vi "Execute.UI.Running.vi"(8 "error in (no error)":errorcluster, 11 "Cluster":T1={"NIVS.BaseLogPath"=path "", "NIVS.SystemDefinitionFile"=path "", "NIVS.Events"={"SequenceEvent"=refnum, "SystemChangeEvent"=refnum, "WorkspaceEvent"=refnum}, "NIVS.SequenceState"=enum."Idle", "NIVS.GatewayIPAddress"="", "NIVS.DataLogSpecRef"=refnum, "NIVS.DataLogManagerRef"=refnum, "NIVS.LogSessionGUID"="", "NIVS.WorkspaceManager"=refnum, "NIVS.Deployed"=FALSE, "NIVS.ProfileRef"=refnum, "NIVS.ProfileCallback"=refnum, "NIVS.SystemStateRefs"={"CustDatRef"=refnum, "EvtRef"=refnum}, "UI.Abort"=refnum, "UI.Pause"=refnum, "UI.EnableLogging"=refnum, "UI.Start"=refnum, "UI.LogChannels"=refnum, "UI.StartIteration"=refnum, "UI.StartStep"=refnum, "UI.Sequence"=refnum, "UI.PreviewMode"=refnum, "UI.Graph"=refnum, "UI.BaseFileName"=refnum, "UI.Profiles"=refnum, "UI.CurrentStep"=refnum, "UI.CurrentIteration"=refnum, "UI.TotalIterations"=refnum, "Sequence.AbortChannel"="", "Sequence.StepInfoChannel"="", "Sequence.Iterations"=0, "Sequence.IterationInfoChannel"="", "Sequence.#ofColumns"=0, "Events.State"=refnum, "Events.Test Result"=refnum, "Events.Progress"=refnum, "INI.Settings"={"Build Location"=path "C:/Simple Sequence Editor/SequenceRepo", "LoggingLocation"=path ""}, "UI.Skip"=refnum, "Sequence.SkipChannel"="", "Restart.Path"=path "", "UI.Duration"=refnum, "Sequence.DurationChannel"=""}) -> (0 "error out":errorcluster)   [LabVIEW 2013, in "Simple Sequence Tools - Execution.lvlib"]
uses:
  Simple Sequence Tools - Execution.lvlib
  Types/Main.StateVariables.ctl
  Types/Execute.UserEventRefs.ctl
  <vilib>/NI Veristand/Execution/Workspace/SystemStateRegEventRef.ctl
  Types/Execution.SequenceState.ctl
  <vilib>/NI Veristand/Execution/DataLogging/DataLoggingSpecification Ref.ctl
  NationalInstruments.VeriStand.ClientAPI
  <vilib>/NI Veristand/Execution/DataLogging/IDataLogging Ref.ctl
  <vilib>/NI Veristand/Execution/Workspace/WorkspaceAPI.ctl
  NationalInstruments.VeriStand.RealTimeSequenceDefinitionApi
  <vilib>/NI Veristand/Execution/Workspace/SystemStateEventRef.ctl
  Shared/Types/INI.Settings
  <vilib>/NI Veristand/Execution/Workspace/NI_VS Workspace ExecutionAPI.lvlib
  <vilib>/NI Veristand/Execution/DataLogging/NI_VS Data Logging API.lvlib
  Shared/Simple Sequence Tools - Shared.lvlib
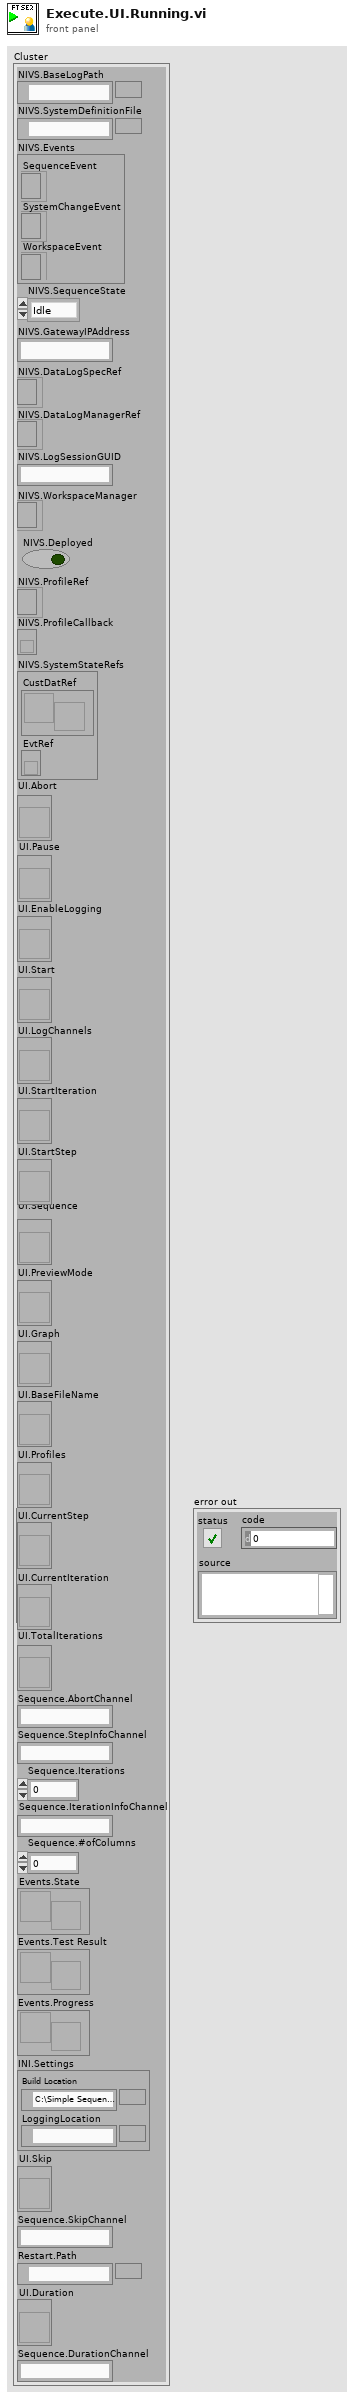
[diagram p1: front panel]
types:
  T1 = typedef "Simple Sequence Tools - Execution.lvlib/Main.StateVariables.ctl" = cluster{"NIVS.BaseLogPath":path, "NIVS.SystemDefinitionFile":path, "NIVS.Events":T2, "NIVS.SequenceState":T4, "NIVS.GatewayIPAddress":string, "NIVS.DataLogSpecRef":T5, "NIVS.DataLogManagerRef":T6, "NIVS.LogSessionGUID":string, "NIVS.WorkspaceManager":T7, "NIVS.Deployed":bool, "NIVS.ProfileRef":refnum<k24>, "NIVS.ProfileCallback":refnum<k27>, "NIVS.SystemStateRefs":T8, "UI.Abort":refnum<vi>, "UI.Pause":refnum<vi>, "UI.EnableLogging":refnum<vi>, "UI.Start":refnum<vi>, "UI.LogChannels":refnum<vi>, "UI.StartIteration":refnum<vi>, "UI.StartStep":refnum<vi>, "UI.Sequence":refnum<vi>, "UI.PreviewMode":refnum<vi>, "UI.Graph":refnum<vi>, "UI.BaseFileName":refnum<vi>, "UI.Profiles":refnum<vi>, "UI.CurrentStep":refnum<vi>, "UI.CurrentIteration":refnum<vi>, "UI.TotalIterations":refnum<vi>, "Sequence.AbortChannel":string, "Sequence.StepInfoChannel":string, "Sequence.Iterations":u32, "Sequence.IterationInfoChannel":string, "Sequence.#ofColumns":i32, "Events.State":refnum<user-event>, "Events.Test Result":refnum<user-event>, "Events.Progress":refnum<user-event>, "INI.Settings":T9, "UI.Skip":refnum<vi>, "Sequence.SkipChannel":string, "Restart.Path":path, "UI.Duration":refnum<vi>, "Sequence.DurationChannel":string}
  T2 = typedef "Simple Sequence Tools - Execution.lvlib/Execute.UserEventRefs.ctl" = cluster{"SequenceEvent":refnum<event-registration>, "SystemChangeEvent":T3, "WorkspaceEvent":refnum<event-registration>}
  T3 = typedef "NI_VS Workspace ExecutionAPI.lvlib/SystemStateRegEventRef.ctl" = refnum<event-registration>
  T4 = typedef "Simple Sequence Tools - Execution.lvlib/Execution.SequenceState.ctl" = enum16{"Idle", "Initializing", "Running", "Paused", "Finalizing", "Complete"}
  T5 = typedef "NI_VS Data Logging API.lvlib/DataLoggingSpecification Ref.ctl" = refnum<k24>
  T6 = typedef "NI_VS Data Logging API.lvlib/IDataLogging Ref.ctl" = refnum<k24>
  T7 = typedef "NI_VS Workspace ExecutionAPI.lvlib/WorkspaceAPI.ctl" = refnum<k24>
  T8 = typedef "NI_VS Workspace ExecutionAPI.lvlib/SystemStateEventRef.ctl" = cluster{"CustDatRef":refnum<user-event>, "EvtRef":refnum<k27>}
  T9 = typedef "Simple Sequence Tools - Shared.lvlib/INI.Settings" = cluster{"Build Location":path, "LoggingLocation":path}
  T10 = enum8{"Enabled", "Disabled", "Disabled and Grayed Out"}
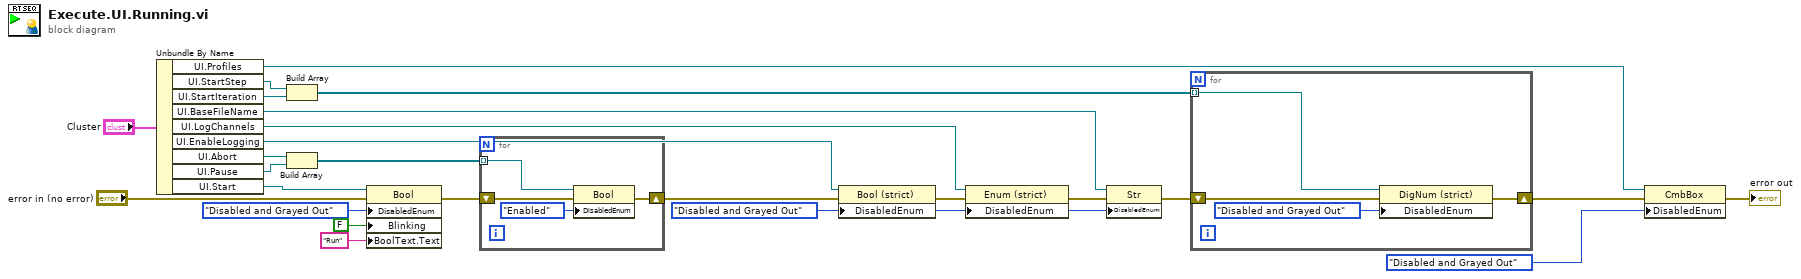
[diagram p0: block diagram]
diagram:
  w7 = T10."Disabled and Grayed Out" ("Disabled")
  n1 = Unbundle By Name("Cluster") -> ("UI.Profiles"=w25:refnum<vi>, "UI.StartStep"=w22:refnum<vi>, "UI.StartIteration"=w21:refnum<vi>, "UI.BaseFileName"=w8:refnum<vi>, "UI.LogChannels"=w19:refnum<vi>, "UI.EnableLogging"=w18:refnum<vi>, "UI.Abort"=w14:refnum<vi>, "UI.Pause"=w15:refnum<vi>, "UI.Start"=w9:refnum<vi>)
  n2 = Build Array(w22, w21) -> (w23:refnum<vi>[])
  n3 = Build Array(w14, w15) -> (w16:refnum<vi>[])
  n4 = property class="Bool"(reference=w9, error in="error in (no error)", "DisabledEnum"=T10."Disabled and Grayed Out" ("Disabled"), "Blinking"=FALSE, "BoolText.Text"="Run" ("Boolean Text.Text")) -> (error out=w10:errorcluster)  [unwired: 1 out]
  n5 = for {
    tunnel: w16 -> [w29] mode=indexing
    shift-right: [w27] -> w17
    shift-left: w10 -> [w26]
    n6 = property class="Bool"(reference=w29, error in=w26, "DisabledEnum"=T10."Enabled" ("Disabled")) -> (error out=w27:errorcluster)  [unwired: 1 out]
  }
  n7 = property class="Bool (strict)"(reference=w18, error in=w17, "DisabledEnum"=w7) -> (error out=w20:errorcluster)  [unwired: 1 out]
  n8 = property class="Enum (strict)"(reference=w19, error in=w20, "DisabledEnum"=w7) -> (error out=w6:errorcluster)  [unwired: 1 out]
  n9 = property class="Str"(reference=w8, error in=w6, "DisabledEnum"=w7) -> (error out=w5:errorcluster)  [unwired: 1 out]
  n10 = for {
    tunnel: w23 -> [w33] mode=indexing
    shift-right: [w31] -> w24
    shift-left: w5 -> [w30]
    n11 = property class="DigNum (strict)"(reference=w33, error in=w30, "DisabledEnum"=T10."Disabled and Grayed Out" ("Disabled")) -> (error out=w31:errorcluster)  [unwired: 1 out]
  }
  n12 = property class="CmbBox"(reference=w25, error in=w24, "DisabledEnum"=T10."Disabled and Grayed Out" ("Disabled")) -> (error out=→"error out":errorcluster)  [unwired: 1 out]
